vi "ExSubSetupCam.vi"(2 "error in (no error)":errorcluster, 3 "Camera Handle":u32) -> (0 "error out":errorcluster, 1 "Camera Handle":u32)   [LabVIEW 2010]
panel:
  # "This is a SubVI that sets the cleans and shutter"
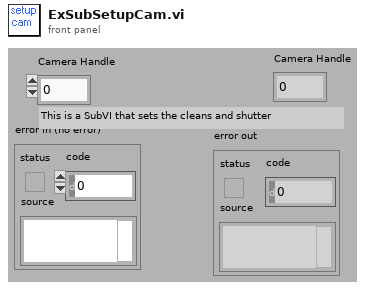
[diagram p1: front panel]
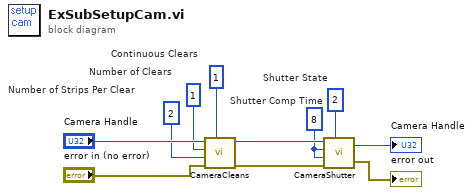
[diagram p0: block diagram]
diagram:
  w2 = u32 1  # Number of Clears
  w1 = u32 2  # Number of Strips Per Clear
  w3 = u32 1  # Continuous Clears
  w4 = u32 2  # Shutter State
  w5 = u32 8  # Shutter Comp Time
  n1 = call <userlib>:"CameraCleans.vi"("Camera Handle"="Camera Handle", "Number of Clears"=w2, "Number of Strips Per Clear"=w1, "error in"="error in (no error)", "Continuous Clears"=w3) -> ("Camera Handle"=w6:u32, "error out"=w7:errorcluster)
  n2 = call <userlib>:"CameraShutter.vi"("Camera Handle"=w6, "Shutter Comp Time: Pre Open"=w5, "Shutter Comp Time: Post Open"=w5, "error in"=w7, "Shutter State"=w4) -> ("Camera Handle"=→"Camera Handle":u32, "error out"=→"error out":errorcluster)
